vi "GetType.vi"(8 "error in (no error)":errorcluster, 11 "Start Scan Msg":refnum<class "Start Scan Msg.lvclass">) -> (0 "error out":errorcluster, 2 "Data Sample":variant, 3 "Start Scan Msg":refnum<class "Start Scan Msg.lvclass">)   [LabVIEW 2015, in "CS++MCS.lvlib" / "Start Scan Msg.lvclass"]
uses:
  Start Scan Msg.lvclass
  Start Scan Msg.lvclass/Start Scan Msg.ctl
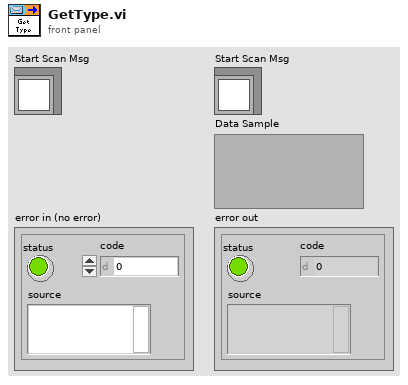
[diagram p1: front panel]
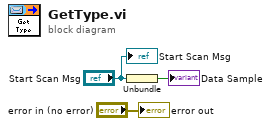
[diagram p0: block diagram]
diagram:
  n1 = Unbundle("Start Scan Msg") -> (→"Data Sample":bool)
  "error out" <- "error in (no error)"
  "Start Scan Msg" <- "Start Scan Msg"
